vi "Write OOB DVR.vi"(8 "error in":errorcluster, 10 "Commands (bitwise)":u64, 11 "OOB in":refnum<class "CIFOutOfBand.lvclass">) -> (0 "error out":errorcluster, 3 "OOB out":refnum<class "CIFOutOfBand.lvclass">)   [LabVIEW 2021, in "CIFOutOfBand.lvclass"]
uses:
  CIFOutOfBand.lvclass
  CIFOutOfBand.lvclass/CIFOutOfBand.ctl
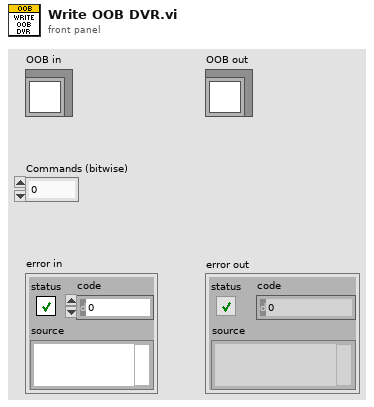
[diagram p1: front panel]
types:
  T1 = typedef "CIFOutOfBand2.lvclass/OOB Container.ctl" = cluster{"Commands":u64, "Payload":variant}
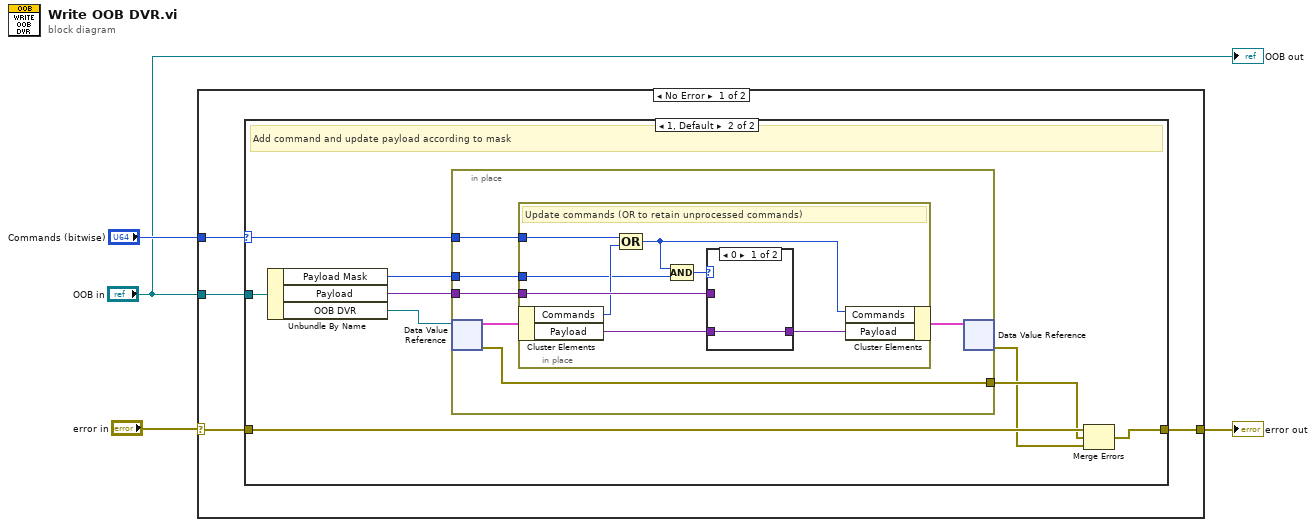
[diagram p0: block diagram]
diagram:
  n1 = case shown="No Error" "error in" {
    selector: "error in" -> [w7 w35]
    tunnel: [w8 w35] -> w3
    tunnel: "OOB in" -> [w6 _]
    tunnel: "Commands (bitwise)" -> [w5 _]
    frame No Error {
      n2 = case shown="1, Default" w5 {
        selector: w5 -> [_ w16]
        tunnel: [w9 w18] -> w8
        tunnel: w7 -> [w9 w17]
        tunnel: w6 -> [_ w10]
        frame 0 {
          # "No Command, skip"
        }
        frame 1, Default {
          # "Add command and update payload according to mask"
          n3 = Unbundle By Name(w10) -> ("Payload Mask"=w11:u64, "Payload"=w12:variant, "OOB DVR"=w13:refnum<data-value>)
          n4 = in-place {
            in-place-border: [w24] -> w15
            in-place-border: w16 -> [w22]
            in-place-border: w12 -> [w20]
            in-place-border: w11 -> [w19]
            n5 = in-place-dvr #1(w13) -> (w23:T1, w24:errorcluster)
            n6 = in-place {
              in-place-border: w22 -> [w28]
              in-place-border: w20 -> [w31]
              in-place-border: w19 -> [w27]
              # "Update commands (OR to retain unprocessed commands)"
              n7 = in-place-cluster #2(w23) -> ("Commands"=w30:u64, "Payload"=w32:variant)
              n8 = Compound Arithmetic op=OR(w28, w30) -> (w25:u64)
              n9 = Compound Arithmetic op=AND(w25, w27) -> (w26:u64)
              n10 = case shown="0" w26 {
                tunnel: w32 -> [w33 _]
                tunnel: [w33 w34] -> w29
                tunnel: w31 -> [_ w34]
                frame 0 {
                }
                frame 1, Default {
                }
              }
              n11 = in-place-cluster #2("Commands"=w25, "Payload"=w29) -> (w21:T1)
            }
            n12 = in-place-dvr #1(w21) -> (w14:errorcluster)  [unwired: 1 out]
          }
          n13 = Merge Errors(w17, w15, w14) -> (w18:errorcluster)
        }
      }
    }
    frame Error {
    }
  }
  "error out" <- w3
  "OOB out" <- "OOB in"
